vi "_RT Correct Ramping Step.vi"(5 "MR Parameters":T1[](array[typedef]), 6 "Ramping Masses":T2[](array[typedef]), 7 "Primary Steps":i32) -> (2 "Ramping Channels":T2[](array[typedef]))   [LabVIEW 2015]
uses:
  Type/_RT Active Ch.ctl
  Type/_Mass Range Parameters.ctl
  _RT Global.vi
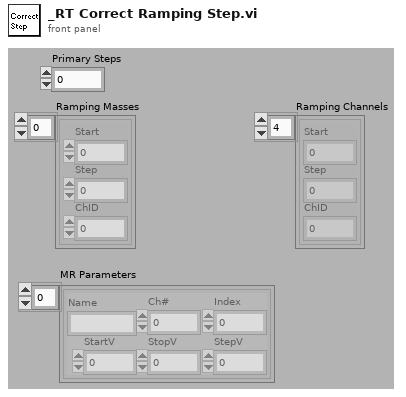
[diagram p1: front panel]
types:
  T1 = typedef "_Mass Range Parameters.ctl" = cluster{"Name":string, "Ch#":u8, "StartV":dbl, "StopV":dbl, "StepV":dbl, "Index":u8}
  T2 = typedef "_RT Active Ch.ctl" = cluster{"Start":i32, "Step":i32, "ChID":i32}
  T3 = typedef "_RT Configuration 2.ctl" = cluster{"Name":string, "Ch#":u8, "Min":dbl, "Max":dbl, "Def+":dbl, "Def-":dbl, "Offset":dbl, "Slope":dbl, "Type":u8, "Description":string, "SettleT":dbl}
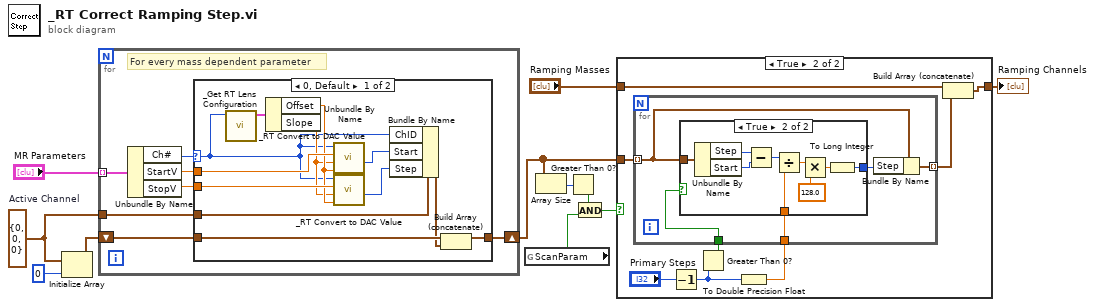
[diagram p0: block diagram]
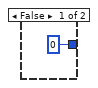
[diagram p4: hidden frame]
diagram:
  w6 = T2 {"Start"=0, "Step"=0, "ChID"=0}  # Active Channel
  n1 = Initialize Array(w6, 0 ("dimension size")) -> (w5:T2[])
  n2 = for {
    tunnel: "MR Parameters" -> [w18] mode=indexing
    tunnel: w6 -> [w15]
    shift-right: [w12] -> w4
    shift-left: w5 -> [w13]
    # "For every mass dependent parameter"
    n3 = Unbundle By Name(w18) -> ("Ch#"=w14:u8, "StartV"=w17:dbl, "StopV"=w16:dbl)
    n4 = case shown="0, Default" w14 {
      selector: w14 -> [w22 _]
      tunnel: w17 -> [w30 _]
      tunnel: w16 -> [w29 _]
      tunnel: w15 -> [w23 _]
      tunnel: w13 -> [w21 w31]
      tunnel: [w19 w31] -> w12
      frame 0, Default {
        n5 = call "_Get RT Lens Configuration.vi"("Channel #"=w22) -> ("Lens Configuration"=w24:T3)  [unwired: 5 in, 1 out]
        n6 = Unbundle By Name(w24) -> ("Offset"=w28:dbl, "Slope"=w27:dbl)
        n7 = call "_RT Convert to DAC Value.vi"("Offset"=w28, "Slop"=w27, "Number"=w30, "Channel"=w22) -> ("DAC Value"=w26:i32)  [unwired: 1 in, 6 out]
        n8 = call "_RT Convert to DAC Value.vi"("Offset"=w28, "Slop"=w27, "Number"=w29, "Channel"=w22) -> ("DAC Value"=w25:i32)  [unwired: 1 in, 6 out]
        n9 = Bundle By Name(cluster=w23, "ChID"=w22, "Start"=w26, "Step"=w25) -> (w20:T2)
        n10 = Build Array (concatenate)(w21, w20) -> (w19:T2[])
      }
      frame 1, 2, 4, 5, 7, 9 {
      }
    }
  }
  n11 = global read "_RT Global.vi" "ScanParam"() -> (w1:bool)
  n12 = Array Size(array=w4) -> (size(s)=w11:i32)
  n13 = Greater Than 0?(x=w11) -> (x > 0?=w3:bool)
  n14 = And(x=w3, y=w1) -> (x .and. y?=w2:bool)
  n15 = case shown="True" w2 {
    tunnel: w4 -> [_ w39]
    tunnel: [w32 w35] -> w9
    tunnel: "Ramping Masses" -> [w32 w37]
    frame False {
    }
    frame True {
      n16 = Decrement(x="Primary Steps") -> (x-1=w34:i32)
      n17 = Greater Than 0?(x=w34) -> (x > 0?=w33:bool)
      n18 = To Double Precision Float(number=w34) -> (double precision float=w38:dbl)
      n19 = for {
        tunnel: w39 -> [w44] mode=indexing
        tunnel: w38 -> [w45]
        tunnel: [w42] -> w36 mode=indexing
        tunnel: w33 -> [w41]
        n20 = case shown="True" w41 {
          tunnel: w45 -> [_ w52]
          tunnel: w44 -> [_ w51]
          tunnel: [0 w50] -> w43
          frame False {
          }
          frame True {
            n21 = Unbundle By Name(w51) -> ("Step"=w55:i32, "Start"=w54:i32)
            n22 = Subtract(x=w55, y=w54) -> (x-y=w53:i32)
            n23 = Divide(x=w53, y=w52) -> (x/y=w49:dbl)
            n24 = Multiply(x=w49, y=128.0) -> (x*y=w47:dbl)
            n25 = To Long Integer(number=w47) -> (32bit integer=w50:i32)
          }
        }
        n26 = Bundle By Name(cluster=w44, "Step"=w43) -> (w42:T2)
      }
      n27 = Build Array (concatenate)(w37, w36) -> (w35:T2[])
    }
  }
  "Ramping Channels" <- w9
